vi "Configure Reference Levels.vi"(0 "VISA Resource Name":refnum<visa-resource-name>, 5 "Low Ref (10.0 %)":dbl=10.0 format="%.2p", 7 "Mid Ref (50.0 %)":dbl=50.0 format="%.2p", 9 "High Ref (90.0 %)":dbl=90.0 format="%.2p", 11 "error in (no error)":errorcluster {"code" format="%.0x"}) -> (4 "VISA Resource Name Out":refnum<visa-resource-name>, 15 "error out":errorcluster {"code" format="%.0x"})   [LabVIEW 2010, in "Tektronix TDS 3000 Series.lvlib"]
doc: "This VI configures the reference levels for waveform measurements. \n\nNotes:\n\n(1) You must call this VI before you call the tktds3k Read Waveform Measurement VI to take a rise time, fall time, width negative, width positive, duty cycle negative, or duty cycle positive measurement."
uses:
  <instrlib>/Tektronix TDS 3000 Series/Tektronix TDS 3000 Series.lvlib
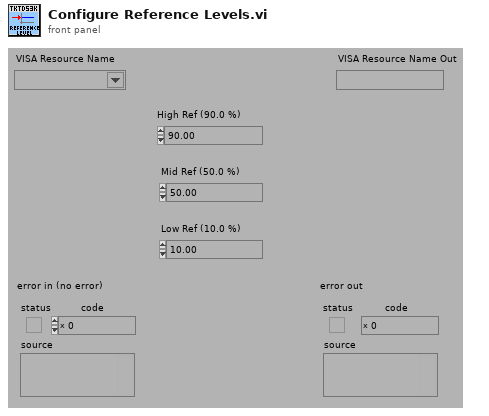
[diagram p1: front panel]
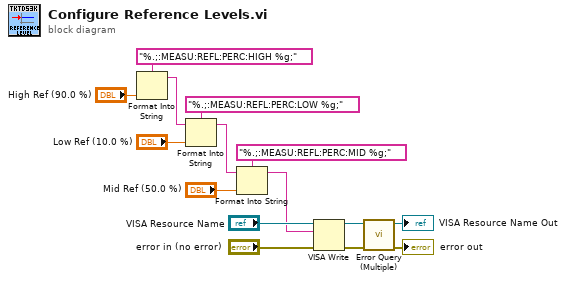
[diagram p0: block diagram]
diagram:
  n1 = Format Into String(format string="%.;:MEASU:REFL:PERC:HIGH %g;", "High Ref (90.0 %)") -> (resulting string=w7:string)  [unwired: 2 in, 1 out]
  n2 = Format Into String(format string="%.;:MEASU:REFL:PERC:LOW %g;", initial string=w7, "Low Ref (10.0 %)") -> (resulting string=w6:string)  [unwired: 1 in, 1 out]
  n3 = Format Into String(format string="%.;:MEASU:REFL:PERC:MID %g;", initial string=w6, "Mid Ref (50.0 %)") -> (resulting string=w5:string)  [unwired: 1 in, 1 out]
  n4 = VISA Write(VISA resource name="VISA Resource Name", write buffer=w5, error in (no error)="error in (no error)") -> (VISA resource name out=w4:refnum<visa-resource-name>, error out=w3:errorcluster)  [unwired: 1 out]
  n5 = call <instrlib>:"Error Query (Multiple).vi"("error in (no error)"=w3, "VISA Resource Name"=w4) -> ("error out"=→"error out":errorcluster, "VISA Resource Name Out"=→"VISA Resource Name Out":refnum<visa-resource-name>)  [unwired: 6 in, 2 out]
